vi "comparison (like if).vi"() -> ()   [LabVIEW 2017]
panel:
  in  "Numeric 2":dbl
  in  "Numeric":dbl
  out "Boolean":bool
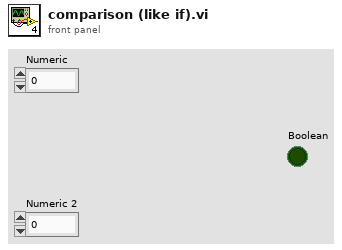
[diagram p1: front panel]
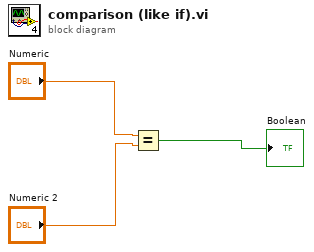
[diagram p0: block diagram]
diagram:
  n1 = Equal?(x="Numeric", y="Numeric 2") -> (x = y?=→"Boolean":bool)
